vi "Post_Process_Results_File.vi"(3 "Top level Folder":path, 4 "Post processed Results folder":path, 5 "Results File to Post Process":path) -> (0 "Error":string, 1 "Files not found":i32, 2 "File Processed":i32)   [LabVIEW 2010]
uses:
  Gen Trav/Multi_Run_Status.ctl
  Controls/Save_Data.ctl
  Controls/Setup.ctl
  Controls/Post_Process.ctl
  Globals/Meas_global.vi
panel:
  out "Current Path":path
  in  "stop":bool
  out "Raw Data Files Processed":i32(slide) scale=0.0..15.0
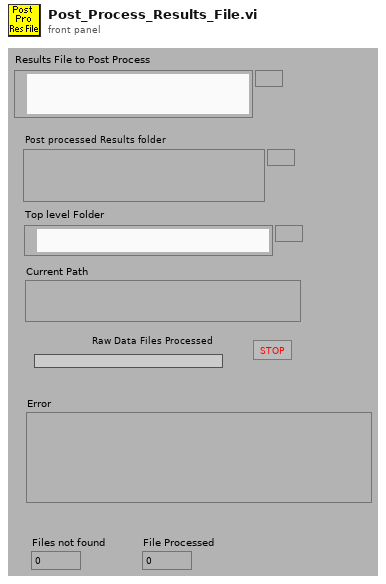
[diagram p1: front panel]
types:
  T1 = typedef "Multi_Run_Status.ctl" = enum16{"Continue", "Jump to Next Point", "Jump to Next Row", "Jump To Fall Back", "Terminate Run"}
  T2 = typedef "Save_Data.ctl" = enum16{"Save No Data", "Save Data"}
  T3 = typedef "Setup.ctl" = enum16{"Run Program", "Show Setup", "Save Current Setup", "Setup Front Panel"}
  T4 = typedef "Post_Process.ctl" = enum16{"Take New Data", "Post Process Raw Data File"}
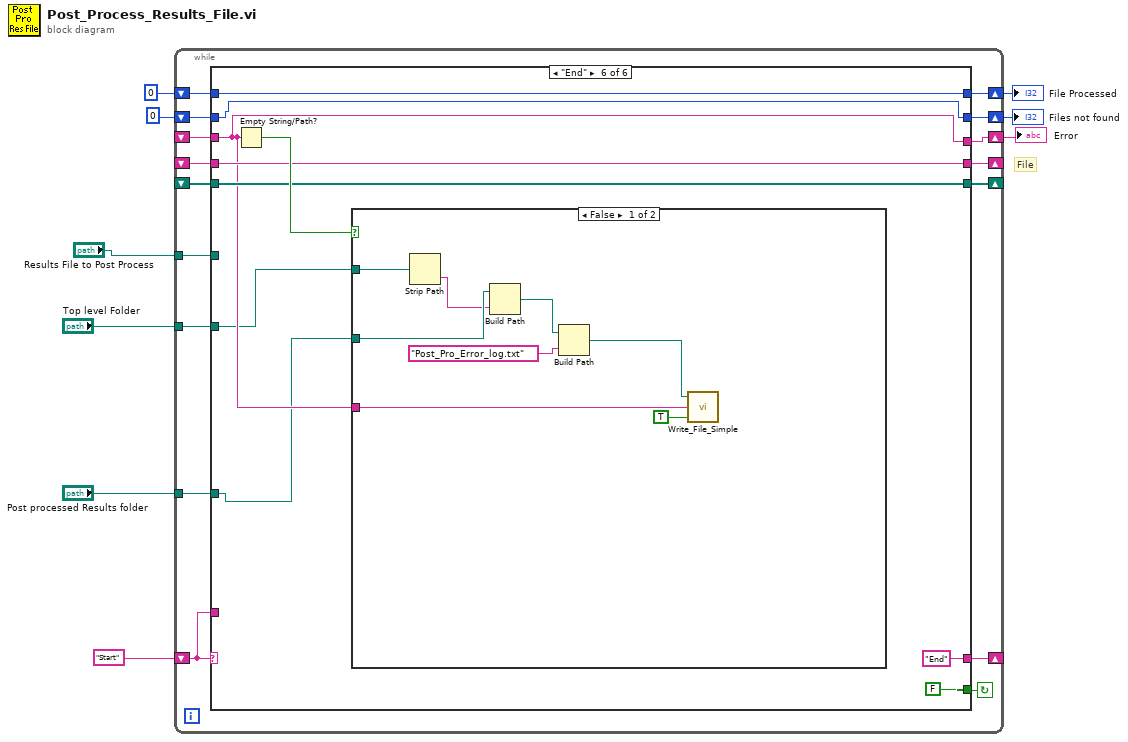
[diagram p0: block diagram]
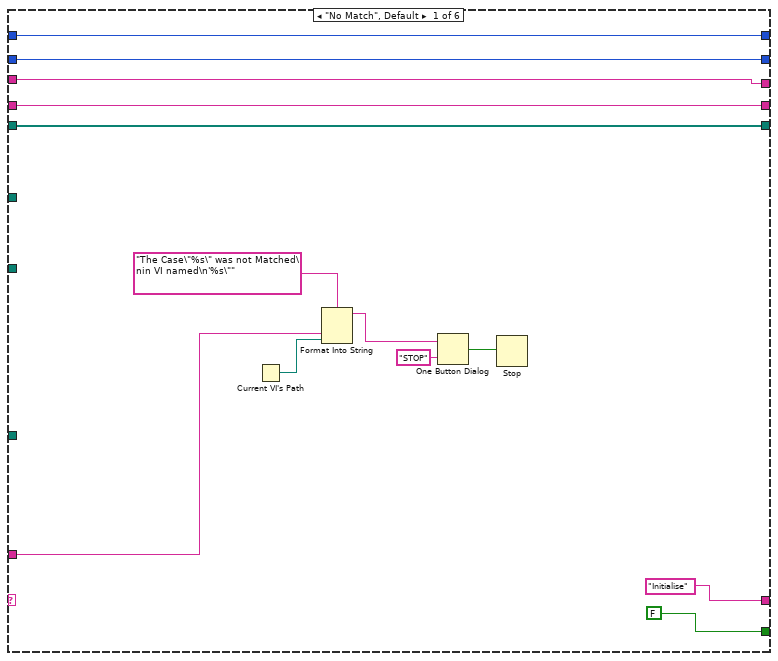
[diagram p2: hidden frame]
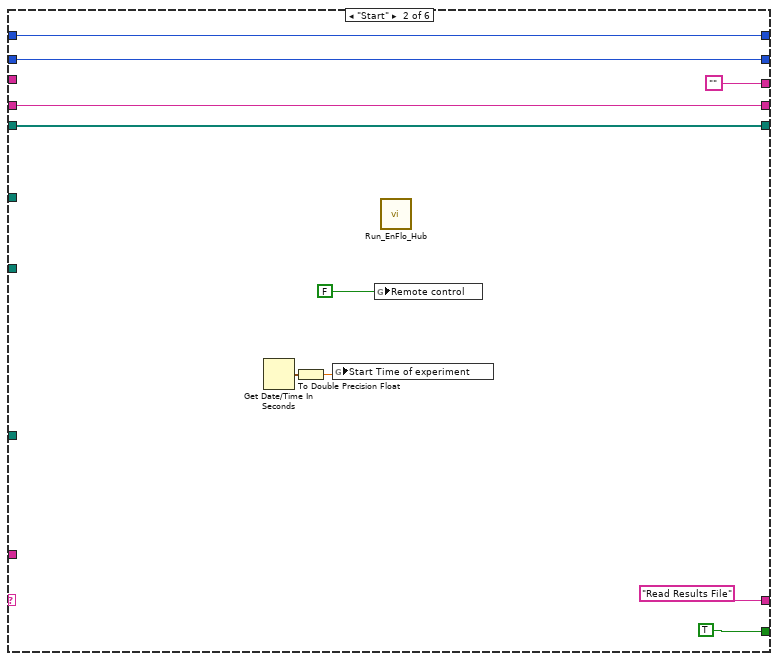
[diagram p3: hidden frame]
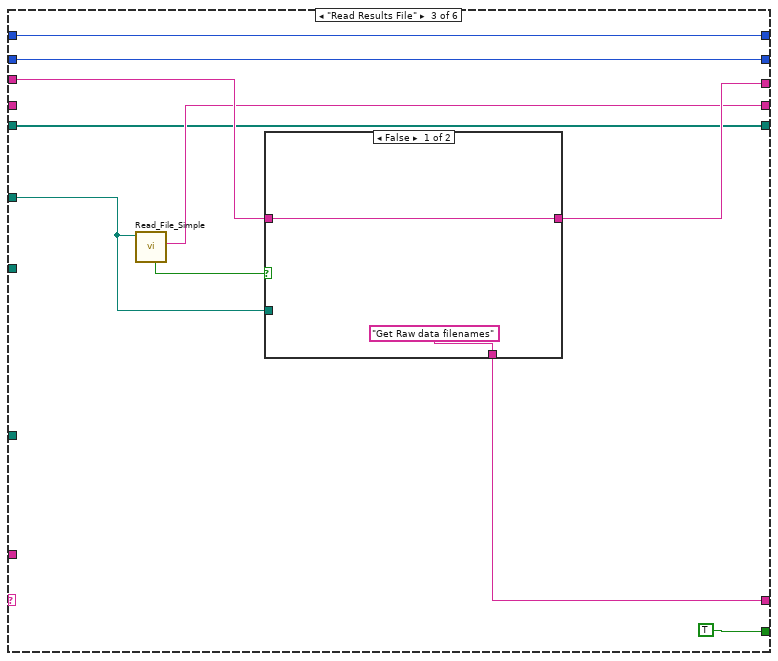
[diagram p4: hidden frame]
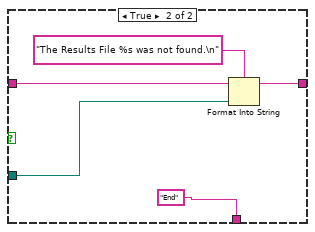
[diagram p5: hidden frame]
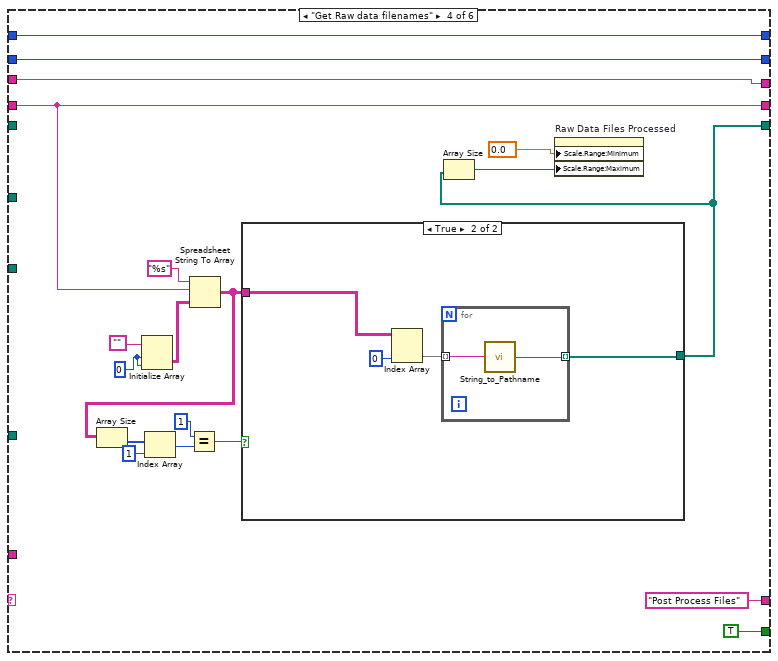
[diagram p6: hidden frame]
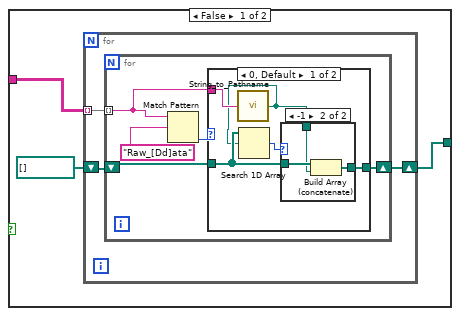
[diagram p7: hidden frame]
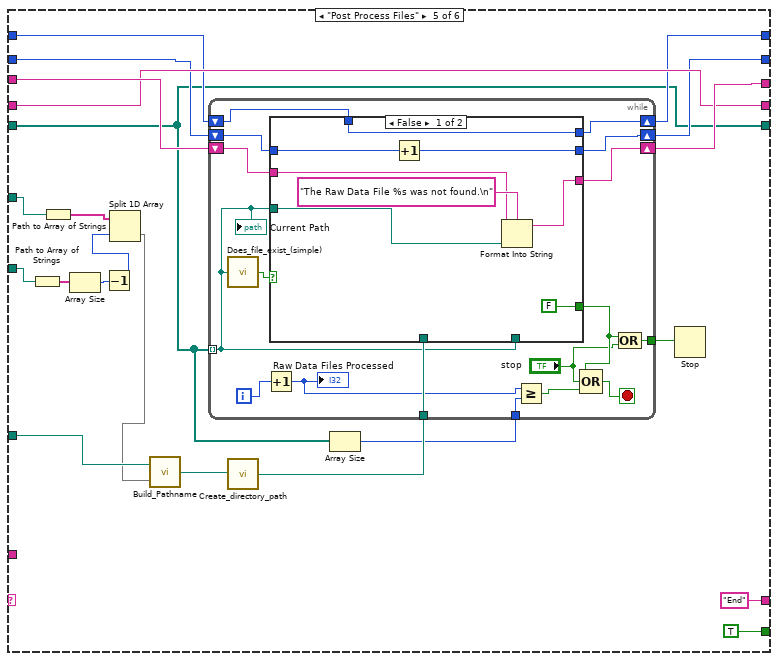
[diagram p10: hidden frame]
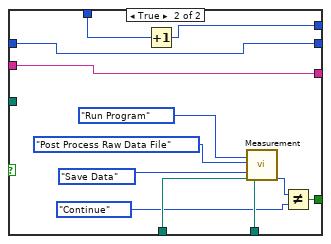
[diagram p11: hidden frame]
diagram:
  # "File"
  n1 = while {
    shift-left: "Start" -> [w23]
    shift-right: [w24] -> _
    tunnel: "Results File to Post Process" -> [w22]
    shift-right: [w21] -> w5
    shift-left: _ -> [w20]
    shift-right: [w19] -> _
    shift-left: _ -> [w18]
    shift-right: [w17] -> _
    shift-left: _ -> [w16]
    tunnel: "Top level Folder" -> [w15]
    tunnel: "Post processed Results folder" -> [w14]
    shift-right: [w12] -> w3
    shift-left: 0 -> [w13]
    shift-right: [w10] -> w1
    shift-left: 0 -> [w11]
    stop <- w25 continue-if-true
    n2 = case shown="\"End\"" w23 {
      tunnel: [FALSE TRUE TRUE TRUE TRUE FALSE] -> w25
      tunnel: ["Initialise" "Read Results File" w53 "Post Process Files" "End" "End"] -> w24
      tunnel: w23 -> [w33 _ _ _ _ _]
      tunnel: w22 -> [_ _ w56 _ w129 _]
      tunnel: [w30 "" w54 w71 w124 w177] -> w21
      tunnel: w20 -> [w30 _ w55 w71 w125 w177]
      tunnel: [w29 w42 w52 w70 w121 w179] -> w19
      tunnel: w18 -> [w29 w42 _ w70 w121 w179]
      tunnel: [w28 w41 w51 w72 w116 w178] -> w17
      tunnel: w16 -> [w28 w41 w51 _ w116 w178]
      tunnel: w15 -> [_ _ _ _ w130 w171]
      tunnel: w14 -> [_ _ _ _ w128 w172]
      tunnel: w13 -> [w26 w39 w49 w66 w120 w173]
      tunnel: [w26 w39 w49 w66 w119 w173] -> w12
      tunnel: w11 -> [w27 w40 w50 w67 w118 w174]
      tunnel: [w27 w40 w50 w67 w117 w174] -> w10
      frame "No Match", Default {
        n3 = Current VI's Path() -> (path=w32:path)
        n4 = Format Into String(format string="The Case\"%s\" was not Matched\nin VI named\n'%s\"" ("Format String"), w33, w32) -> (resulting string=w36:string)  [unwired: 2 in, 1 out]
        n5 = One Button Dialog(message=w36, button name ("OK")="STOP") -> (true=w34:bool)
        n6 = Stop(stop? (T)=w34) -> ()
      }
      frame "Start" {
        n7 = Get Date/Time In Seconds() -> (seconds since 1Jan1904=w46:timestamp)
        n8 = To Double Precision Float(number=w46) -> (double precision float=w45:dbl)
        n9 = global write "Meas_global.vi" "Start Time of experiment"(w45) -> ()
        n10 = global write "Meas_global.vi" "Remote control"(FALSE ("Remote control")) -> ()
        n11 = call "Run_EnFlo_Hub.vi"() -> ()  [unwired: 8 out]
      }
      frame "Read Results File" {
        n12 = call "Read_File_Simple.vi"("Filename"=w56) -> ("Error?"=w57:bool, "string"=w52:string)  [unwired: 2 in, 6 out]
        n13 = case shown="False" w57 {
          tunnel: w56 -> [_ w65]
          tunnel: w55 -> [w60 w63]
          tunnel: [w60 w62] -> w54
          tunnel: ["Get Raw data filenames" "End"] -> w53
          frame False {
          }
          frame True {
            n14 = Format Into String(format string="The Results File %s was not found.\n", initial string=w63, w65) -> (resulting string=w62:string)  [unwired: 1 in, 1 out]
          }
        }
      }
      frame "Get Raw data filenames" {
        w78 = 0 ("Dimension Size")
        n15 = Initialize Array("", w78, w78) -> (w76:string[][])
        n16 = Spreadsheet String To Array(format string="%s", spreadsheet string=w70, array type (2D Dbl)=w76) -> (array=w79:string[][])  [unwired: 1 out]
        n17 = Array Size(array=w79) -> (size(s)=w80:i32[])
        n18 = Index Array(array=w80, index=1) -> (element=w82:i32)
        n19 = Equal?(x=1, y=w82) -> (x = y?=w84:bool)
        n20 = case shown="True" w84 {
          tunnel: w79 -> [w87 w109]
          tunnel: [w86 w106] -> w72
          frame False {
            n21 = for {
              tunnel: w87 -> [w90] mode=indexing
              shift-right: [w88] -> w86
              shift-left: path[] [] -> [w89]
              n22 = for {
                tunnel: w90 -> [w92] mode=indexing
                shift-right: [w91] -> w88
                shift-left: w89 -> [w93]
                n23 = Match Pattern(string=w92, regular expression="Raw_[Dd]ata") -> (offset past match=w94:i32)  [unwired: 4 out]
                n24 = case shown="0, Default" w94 {
                  tunnel: w93 -> [w98 w105]
                  tunnel: w92 -> [w99 _]
                  tunnel: [w100 w105] -> w91
                  frame 0, Default {
                    n25 = call "String_to_Pathname.vi"("Input String"=w99) -> ("path"=w97:path)
                    n26 = Search 1D Array(1D array=w98, element=w97) -> (index of element=w96:i32)  [unwired: 1 out]
                    n27 = case shown="-1" w96 {
                      tunnel: w98 -> [w101 w104]
                      tunnel: [w101 w103] -> w100
                      tunnel: w97 -> [_ w102]
                      frame 0, Default {
                      }
                      frame -1 {
                        n28 = Build Array (concatenate)(w104, w102) -> (w103:path[])
                      }
                    }
                  }
                  frame -1 {
                  }
                }
              }
            }
          }
          frame True {
            n29 = Index Array(array=w109, index (col)=0 ("disabled index (col)")) -> (element=w107:string[])  [unwired: 1 in]
            n30 = for {
              tunnel: w107 -> [w111] mode=indexing
              tunnel: [w110] -> w106 mode=indexing
              n31 = call "String_to_Pathname.vi"("Input String"=w111) -> ("path"=w110:path)
            }
          }
        }
        n32 = Array Size(array=w72) -> (size(s)=w74:i32)
        n33 = property on="Raw Data Files Processed" class="Slide (strict)"("Scale.Range:Minimum"=0.0 ("Write Attribute"), "Scale.Range:Maximum"=w74) -> ()  [unwired: 2 in, 2 out]
      }
      frame "Post Process Files" {
        n34 = Path to Array of Strings(0:w130) -> (2:w133:string[])  [unwired: 1 out]
        n35 = Path to Array of Strings(0:w129) -> (2:w131:string[])  [unwired: 1 out]
        n36 = Array Size(array=w133) -> (size(s)=w132:i32)
        n37 = Decrement(x=w132) -> (x-1=w114:i32)
        n38 = Split 1D Array(array=w131, index=w114) -> (second subarray=w112:string[])  [unwired: 1 out]
        n39 = call "Build_Pathname.vi"("Output Array"=w112, "Pathname"=w128) -> ("Appended path"=w127:path)
        n40 = call "Create_directory_path.vi"("Path name"=w127) -> ("Path name Out"=w126:path)
        n41 = Array Size(array=w116) -> (size(s)=w115:i32)
        n42 = while {
          tunnel: w116 -> [w147] mode=indexing
          tunnel: w126 -> [w149]
          shift-right: [w145] -> w124
          shift-left: w125 -> [w146]
          shift-right: [w143] -> w119
          shift-left: w120 -> [w144]
          shift-right: [w141] -> w117
          shift-left: w118 -> [w142]
          tunnel: w115 -> [w139]
          tunnel: [w134] -> w113
          i -> [w150]
          stop <- w137 stop-if-true
          n43 = call "Does_file_exist_(simple).vi"("Pathname"=w147) -> ("exists?"=w148:bool)
          n44 = Increment(x=w150) -> (x+1=w140:i32)
          "Raw Data Files Processed" <- w140
          n45 = case shown="False" w148 {
            tunnel: w149 -> [_ w168]
            tunnel: w147 -> [_ w167]
            tunnel: w147 -> [w157 _]
            tunnel: w146 -> [w156 w166]
            tunnel: [w155 w166] -> w145
            tunnel: w144 -> [w154 w162]
            tunnel: [w153 w162] -> w143
            tunnel: w142 -> [w152 w164]
            tunnel: [w152 w163] -> w141
            tunnel: [FALSE w159] -> w136
            frame False {
              n46 = Increment(x=w154) -> (x+1=w153:i32)
              n47 = Format Into String(format string="The Raw Data File %s was not found.\n", initial string=w156, w157) -> (resulting string=w155:string)  [unwired: 1 in, 1 out]
            }
            frame True {
              n48 = Increment(x=w164) -> (x+1=w163:i32)
              n49 = call "Measurement.vi"("setup"=Setup."Run Program", "Post Process"=Post_Process."Post Process Raw Data File", "File"=Save_Data."Save Data", "Results file"=w168, "Raw data file"=w167) -> ("Status Out"=w161:T1)  [unwired: 2 in, 12 out]
              n50 = Not Equal?(x=w161, y=Multi_Run_Status."Continue" ("Status Out")) -> (x != y?=w159:bool)
            }
          }
          n51 = Greater Or Equal?(x=w140, y=w139) -> (x >= y?=w138:bool)
          n52 = Compound Arithmetic op=OR(w136, "stop", w138) -> (w137:bool)
          n53 = Compound Arithmetic op=OR(w136, "stop") -> (w134:bool)
          "Current Path" <- w147
        }
        n54 = Stop(stop? (T)=w113) -> ()
      }
      frame "End" {
        n55 = Empty String/Path?(string/path=w177) -> (empty?=w180:bool)
        n56 = case shown="False" w180 {
          tunnel: w172 -> [w183 _]
          tunnel: w177 -> [w187 _]
          tunnel: w171 -> [w184 _]
          frame False {
            n57 = Strip Path(path=w184) -> (name=w182:string)  [unwired: 1 out]
            n58 = Build Path(base path=w183, name or relative path=w182) -> (appended path=w181:path)
            n59 = Build Path(base path=w181, name or relative path="Post_Pro_Error_log.txt" ("string")) -> (appended path=w188:path)
            n60 = call "Write_File_Simple.vi"("append to file? (new file:F)"=TRUE, "character string"=w187, "file path"=w188) -> ()  [unwired: 2 out]
          }
          frame True {
          }
        }
      }
    }
  }
  "Error" <- w5
  "Files not found" <- w3
  "File Processed" <- w1
